vi "Picture to IMAQ.vi"(8 "Error In":errorcluster, 11 "picture":picture) -> (0 "Error Out":errorcluster, 3 "Image":T1(plugin-control))   [LabVIEW 2016]
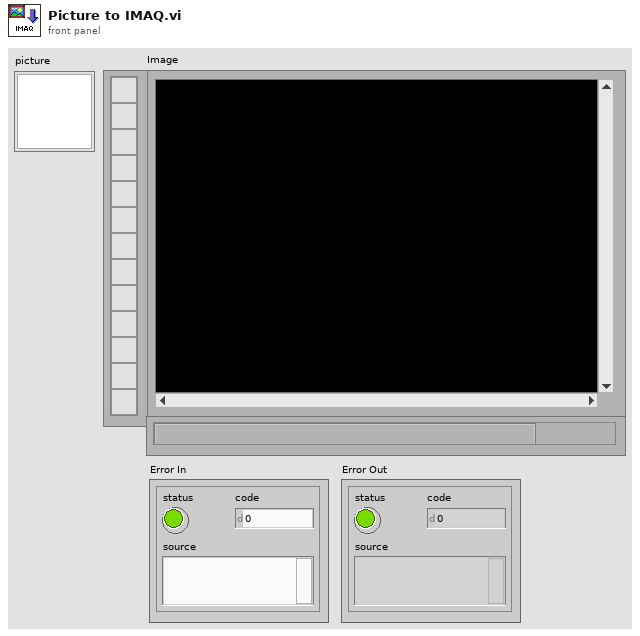
[diagram p1: front panel]
types:
  T1 = typedef "IMAQ Image.ctl" = refnum<image>
  T2 = typedef "Image Type" = u32
  T3 = typedef "imagedata.ctl" = cluster{"image type":i32, "image depth":i32, "image":u8[], "mask":u8[], "colors":u32[], "Rectangle":cluster{"left":i16, "top":i16, "right":i16, "bottom":i16}}
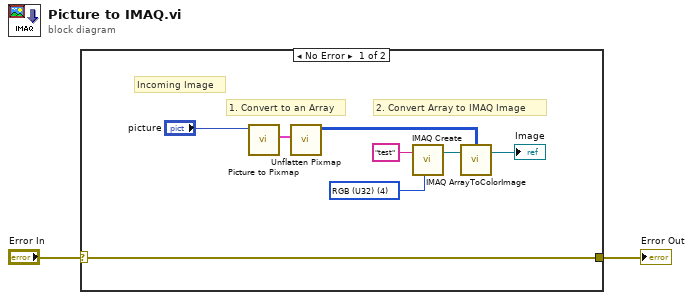
[diagram p0: block diagram]
diagram:
  n1 = case shown="No Error" "Error In" {
    selector: "Error In" -> [w3 w11]
    tunnel: [w3 w11] -> w1
    frame No Error {
      w6 = T2 4 items=["Grayscale (U8)", "Grayscale (I16)", "Grayscale (SGL)", "Complex (CSG)", "RGB (U32)", "HSL (U32)", "RGB (U64)", "Grayscale (U16)"] ("Image Type")
      # "2. Convert Array to IMAQ Image"
      # "1. Convert to an Array"
      # "Incoming Image"
      n2 = call <vilib>:"Picture to Pixmap.vi"("picture"="picture") -> ("image data"=w10:T3)  [unwired: 9 in, 1 out]
      n3 = call <vilib>:"Unflatten Pixmap.vi"("image data"=w10) -> ("24-bit pixmap"=w5:u32[][])  [unwired: 4 in, 6 out]
      n4 = call "IMAQ Create"("Image Name"="test", "Image Type"=w6) -> ("New Image"=w8:T1)  [unwired: 3 in, 1 out]
      n5 = call "IMAQ ArrayToColorImage"("Image Pixels (U32)"=w5, "Image"=w8) -> ("Image Out"=→"Image":T1)  [unwired: 3 in, 1 out]
    }
    frame Error {
    }
  }
  "Error Out" <- w1
